vi "Configure Trigger Source.vi"(8 "error in (no error)":errorcluster, 9 "External Level":dbl, 10 "Trigger Source":enum16{"Immediate", "External"}(ring), 11 "SA-ESA in":refnum<class "SA-ESA.lvclass">) -> (0 "error out":errorcluster, 3 "SA-ESA out":refnum<class "SA-ESA.lvclass">)   [LabVIEW 2020, in "SA-ESA.lvclass"]
uses:
  SA-ESA.lvclass
  C:/Sandbox/Git_Sandbox/WiSpry Test Framework source code (LV20)/WiSpry Test Framework/Instruments/Instrument.lvclass
  Instrument.lvclass/Instrument.ctl
  Instrument.lvclass
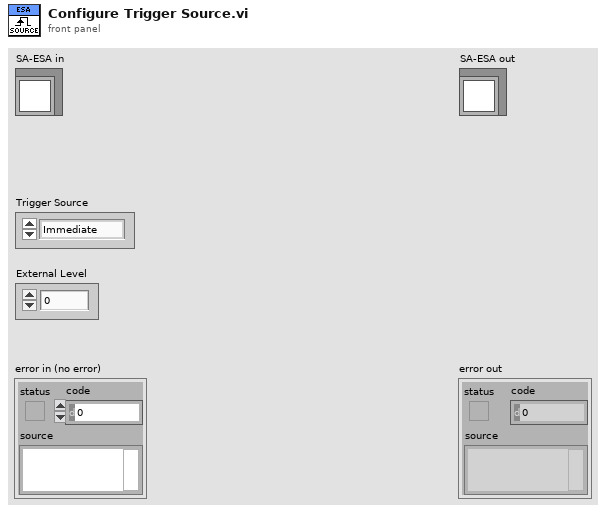
[diagram p1: front panel]
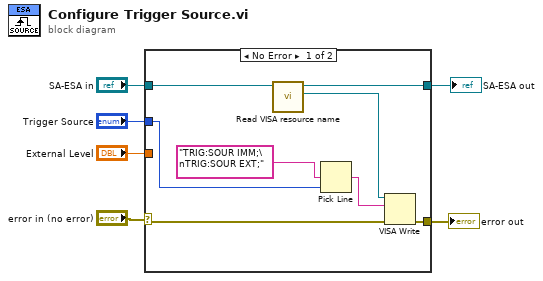
[diagram p0: block diagram]
diagram:
  n1 = case shown="No Error" "error in (no error)" {
    selector: "error in (no error)" -> [w9 w15]
    tunnel: "SA-ESA in" -> [w12 w16]
    tunnel: "Trigger Source" -> [w13 _]
    tunnel: "External Level" -> [_ _]
    tunnel: [w10 w16] -> w1
    tunnel: [w7 w15] -> w2
    frame No Error {
      n2 = call "Read VISA resource name.vi"("Instrument in"=w12) -> ("VISA resource name"=w11:refnum<visa-resource-name>, "Instrument out"=w10:refnum<class "SA-ESA.lvclass">)  [unwired: 9 in]
      n3 = Pick Line(multi-line string="TRIG:SOUR IMM;\nTRIG:SOUR EXT;", line index=w13) -> (output string=w8:string)  [unwired: 1 in]
      n4 = VISA Write(VISA resource name=w11, write buffer=w8, error in (no error)=w9) -> (error out=w7:errorcluster)  [unwired: 2 out]
    }
    frame Error {
    }
  }
  "error out" <- w2
  "SA-ESA out" <- w1
